vi "Channel_mapping_64_BaseOnly.vi"(7 "Base_Ch":i32=16, 11 "Channel IN":i32=16) -> (3 "Operating \nChannel(s)":bool[][](array[boolean]))   [LabVIEW 2023]
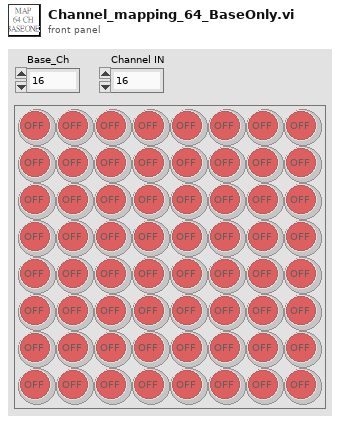
[diagram p1: front panel]
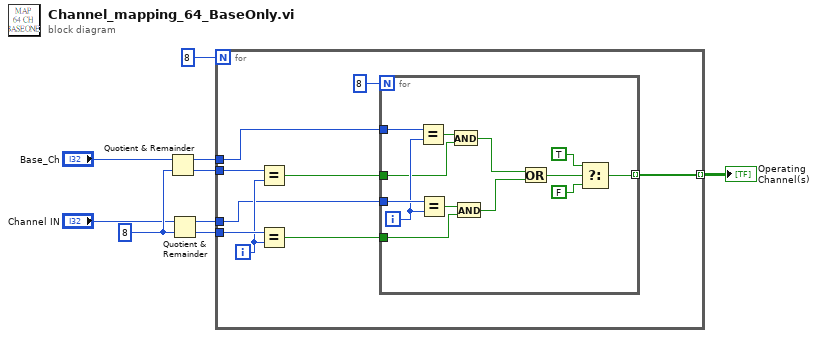
[diagram p0: block diagram]
diagram:
  w5 = 8 ("y")
  n1 = Quotient & Remainder(x="Base_Ch", y=w5) -> (x-y*floor(x/y)=w4:i32, floor(x/y)=w3:i32)
  n2 = Quotient & Remainder(x="Channel IN", y=w5) -> (x-y*floor(x/y)=w6:i32, floor(x/y)=w7:i32)
  n3 = for {
    N: 8 -> [_]
    tunnel: [w17] -> w8 mode=indexing
    tunnel: w7 -> [w16]
    tunnel: w6 -> [w12]
    tunnel: w4 -> [w13]
    tunnel: w3 -> [w15]
    i -> [w14]
    n4 = Equal?(x=w15, y=w14) -> (x = y?=w11:bool)
    n5 = Equal?(x=w16, y=w14) -> (x = y?=w10:bool)
    n6 = for {
      N: 8 -> [_]
      tunnel: [w26] -> w17 mode=indexing
      tunnel: w10 -> [w21]
      tunnel: w13 -> [w31]
      tunnel: w12 -> [w30]
      tunnel: w11 -> [w24]
      i -> [w29]
      n7 = Equal?(x=w31, y=w29) -> (x = y?=w23:bool)
      n8 = Equal?(x=w30, y=w29) -> (x = y?=w22:bool)
      n9 = And(x=w23, y=w24) -> (x .and. y?=w20:bool)
      n10 = And(x=w22, y=w21) -> (x .and. y?=w19:bool)
      n11 = Or(x=w20, y=w19) -> (x .or. y?=w25:bool)
      n12 = Select(t=TRUE, s=w25, f=FALSE) -> (s? t:f=w26:bool)
    }
  }
  "Operating \nChannel(s)" <- w8
